vi "Reset Output Protection.vi"(8 "error in (no error)":errorcluster {"code" format="%.0x"}, 10 "Channel Name (1)":string="1", 11 "VISA resource name":refnum<visa-resource-name>) -> (0 "error out":errorcluster {"code" format="%.0x"}, 3 "VISA resource name out":refnum<visa-resource-name>)   [LabVIEW 2014, in "Agilent N6700 Series.lvlib"]
doc: "Resets the power supply's output protection after an over-voltage, over-current, or other output protection condition occurs.\n\nAn over-voltage condition occurs when the output voltage is equal to or greater than the value of Limit in <B>Configure Over Voltage Protection.vi</B>. \n\nAn over-current condition occurs when the output current is equal to or greater than the value of Limit in <B>Configure Current Limit.vi</B> and Behavior in <B>Configure Current Limit.vi</B> is set to Trip Limit.\n\nWhen either an over-voltage condition or an over-current condition occurs, the output protection of the power supply disables the output. Once the output protection is reset, the power supply resumes generating a power signal.\n\nYou use <B>Query Output State.vi</B> to determine if the power supply is in an output-protection state."
uses:
  Agilent N6700 Series.lvlib
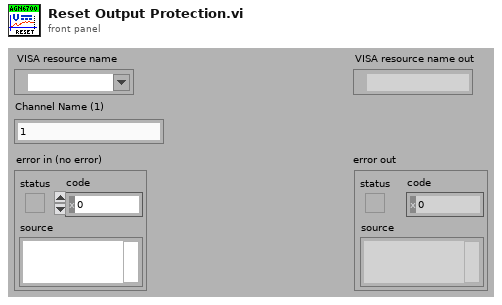
[diagram p1: front panel]
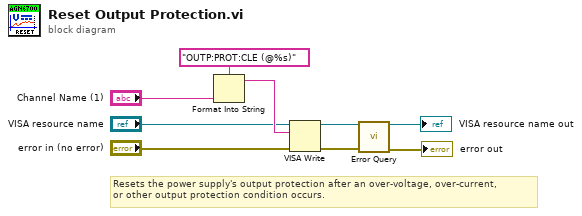
[diagram p0: block diagram]
diagram:
  # "Resets the power supply's output protection after an over-voltage, over-current, \nor other output protection condition occurs."
  n1 = Format Into String(format string="OUTP:PROT:CLE (@%s)", "Channel Name (1)") -> (resulting string=w9:string)  [unwired: 2 in, 1 out]
  n2 = VISA Write(VISA resource name="VISA resource name", write buffer=w9, error in (no error)="error in (no error)") -> (VISA resource name out=w2:refnum<visa-resource-name>, error out=w1:errorcluster)  [unwired: 1 out]
  n3 = call "Error Query.vi"("VISA resource name"=w2, "error in (no error)"=w1) -> ("VISA resource name out"=→"VISA resource name out":refnum<visa-resource-name>, "error out"=→"error out":errorcluster)  [unwired: 10 in, 2 out]
